vi "未命名 1.vi"() -> ()   [LabVIEW 2014]
panel:
  out "数值":i32
  out "错误输出":errorcluster
  out "写入的字节":i32
  out "数据输出":string
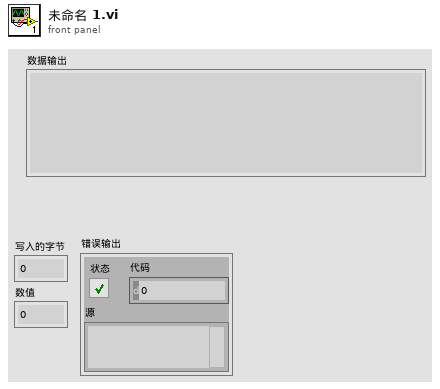
[diagram p1: front panel]
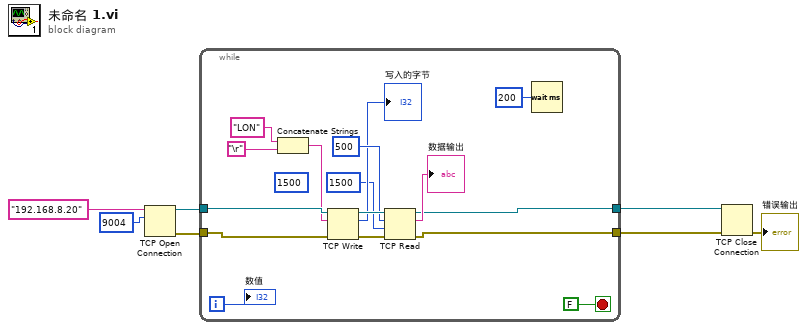
[diagram p0: block diagram]
diagram:
  n1 = TCP Open Connection(address="192.168.8.20" ("地址"), remote port or service name=u16 9004 ("远程端口或服务名称")) -> (connection ID=w4:refnum<k5>, error out=w5:errorcluster)  [unwired: 3 in]
  n2 = while {
    tunnel: w4 -> [w22]
    tunnel: [w14] -> w3
    tunnel: w5 -> [w23]
    tunnel: [w13] -> w2
    i -> [w8]
    stop <- FALSE stop-if-true
    (unwired) 1500 ("超时毫秒(25000)")
    n3 = Concatenate Strings("LON", "\r") -> (w19:string)
    n4 = TCP Write(connection ID=w22, data in=w19, error in (no error)=w23) -> (connection ID out=w18:refnum<k5>, bytes written=→"写入的字节":i32, error out=w17:errorcluster)  [unwired: 1 in]
    n5 = TCP Read(connection ID=w18, bytes to read=500 ("读取的字节"), error in (no error)=w17, 9:1500 ("超时毫秒(25000)")) -> (connection ID out=w14:refnum<k5>, data out=→"数据输出":string, error out=w13:errorcluster)  [unwired: 1 in]
    n6 = Wait (ms)(milliseconds to wait=u32 200 ("等待时间（毫秒）")) -> ()  [unwired: 1 out]
    "数值" <- w8
  }
  n7 = TCP Close Connection(connection ID=w3, error in (no error)=w2) -> (error out=→"错误输出":errorcluster)  [unwired: 1 in, 1 out]
